vi "createFileInstance.vi"(0 "reference in":refnum<class "File Controller.lvclass">, 2 "TSR?":bool, 3 "TYPE:":string, 5 "error in (no error)":errorcluster) -> (14 "reference out":refnum<class "File Controller.lvclass">, 19 "error out":errorcluster)   [LabVIEW 2015, in "File Controller.lvclass"]
uses:
  File Controller.lvclass
  APP/excelFile_class/fileType.ctl
  APP/excelFile_class/excelFile.lvclass
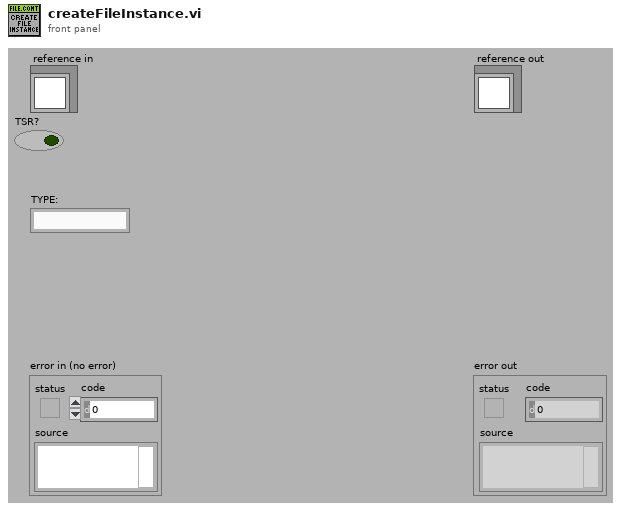
[diagram p1: front panel]
types:
  T1 = typedef "excelFile.lvclass/fileType.ctl" = enum16{"devices", "items", "partsTracking", "TSR"}
  T2 = typedef "File Controller.lvclass/ObjectAttributesRef.ctl" = refnum<data-value>
  T3 = typedef "File Controller.lvclass/ObjectAttributes.ctl" = cluster{"MyAttribute":dbl, "excelFile_refs":refnum<class "excelFile.lvclass">[], "filePaths":path[], "outlookTemplatePaths":path[], "attachmentTemplatePaths":path[], "configFilePath":path, "not_setting":bool[], "python_ref":refnum<class "python.lvclass">, "TSR":cluster{"number":string, "TSR_path":path, "service_path":path}}
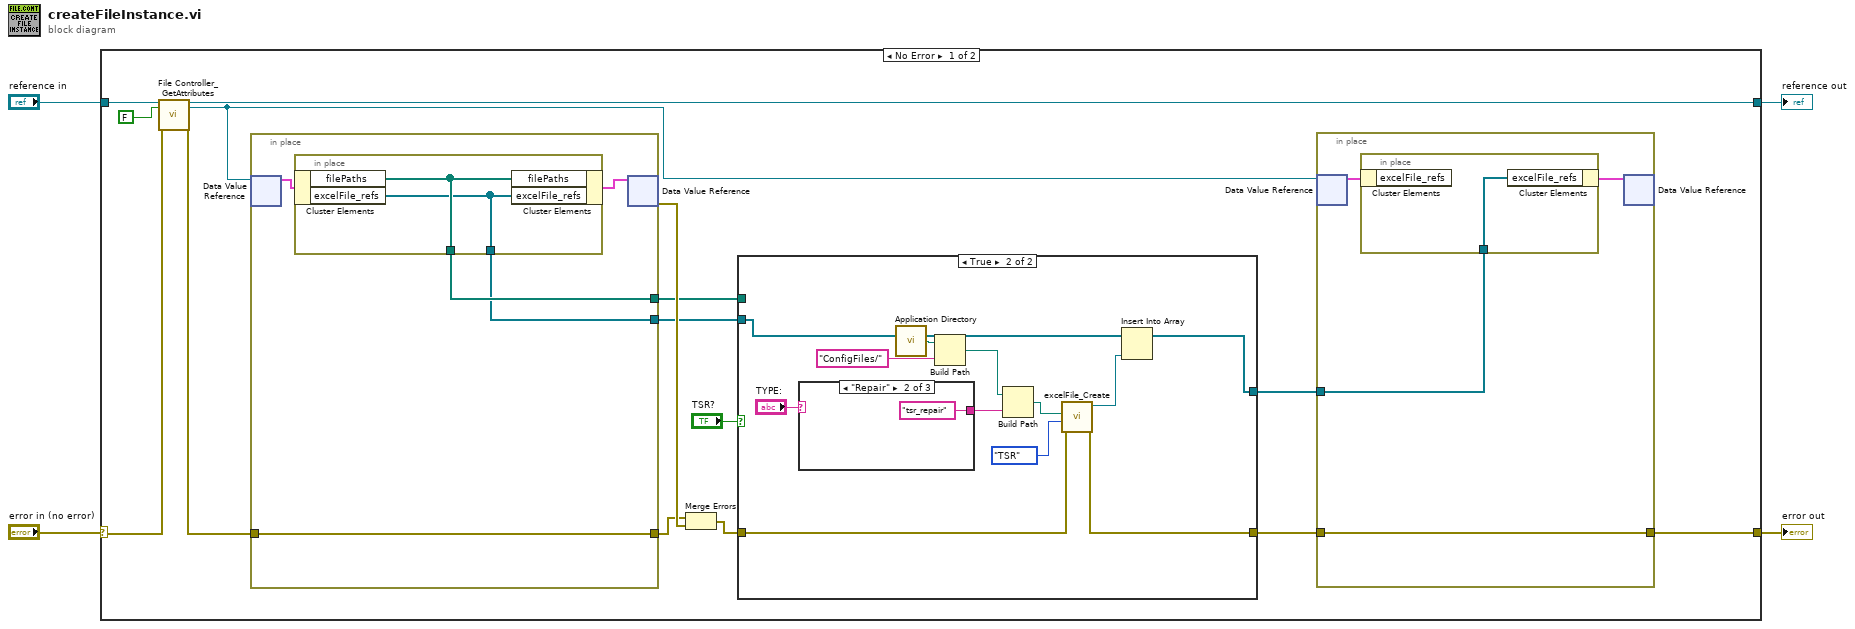
[diagram p0: block diagram]
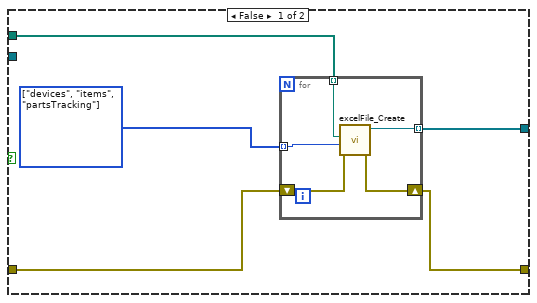
[diagram p2: hidden frame]
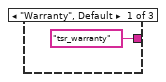
[diagram p3: hidden frame]
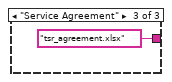
[diagram p4: hidden frame]
diagram:
  n1 = case shown="No Error" "error in (no error)" {
    selector: "error in (no error)" -> [w15 w58]
    tunnel: [w9 w58] -> w3
    tunnel: [w13 w57] -> w1
    tunnel: "reference in" -> [w17 w57]
    frame No Error {
      n2 = call "File Controller_GetAttributes.vi"("reference in"=w17, "return data? (T)"=FALSE, "error in (no error)"=w15) -> ("reference out"=w13:refnum<class "File Controller.lvclass">, "attributes ref"=w8:T2, "error out"=w14:errorcluster)  [unwired: 13 in, 1 out]
      n3 = in-place {
        in-place-border: w14 -> [w52]
        in-place-border: [w52] -> w18
        in-place-border: [w51] -> w11
        in-place-border: [w50] -> w5
        n4 = in-place-dvr #1(w8) -> (w53:T3)  [unwired: 1 out]
        n5 = in-place {
          in-place-border: [w56] -> w51
          in-place-border: [w55] -> w50
          n6 = in-place-cluster #2(w53) -> ("filePaths"=w56:path[], "excelFile_refs"=w55:refnum<class "excelFile.lvclass">[])
          n7 = in-place-cluster #2("filePaths"=w56, "excelFile_refs"=w55) -> (w54:T3)
        }
        n8 = in-place-dvr #1(w54) -> (w19:errorcluster)  [unwired: 1 out]
      }
      n9 = Merge Errors(w18, w19) -> (w12:errorcluster)
      n10 = case shown="True" "TSR?" {
        tunnel: w12 -> [w23 w38]
        tunnel: w11 -> [w22 _]
        tunnel: [w21 w37] -> w10
        tunnel: [w20 w40] -> w7
        tunnel: w5 -> [_ w41]
        frame False {
          w24 = T1[] [enum."devices", enum."items", enum."partsTracking"] items=["devices", "items", "partsTracking", "TSR"]
          n11 = for {
            shift-right: [w26] -> w21
            shift-left: w23 -> [w29]
            tunnel: w24 -> [w28] mode=indexing
            tunnel: w22 -> [w27] mode=indexing
            tunnel: [w25] -> w20 mode=indexing
            n12 = call "excelFile_Create.vi"("error in (no error)"=w29, "fileType"=w28, "Path"=w27) -> ("error out"=w26:errorcluster, "reference out"=w25:refnum<class "excelFile.lvclass">)  [unwired: 7 in]
          }
        }
        frame True {
          n13 = case shown="\"Repair\"" "TYPE:" {
            tunnel: ["tsr_warranty" ("name or relative path") "tsr_repair" ("name or relative path") "tsr_agreement.xlsx" ("name or relative path")] -> w34
            frame "Warranty", Default {
            }
            frame "Repair" {
            }
            frame "Service Agreement" {
            }
          }
          n14 = call <vilib>:"Application Directory.vi"() -> ("Application Directory"=w31:path)
          n15 = Build Path(base path=w31, name or relative path="ConfigFiles/") -> (appended path=w33:path)
          n16 = Build Path(base path=w33, name or relative path=w34) -> (appended path=w30:path)
          n17 = call "excelFile_Create.vi"("error in (no error)"=w38, "fileType"=fileType."TSR", "Path"=w30) -> ("error out"=w37:errorcluster, "reference out"=w39:refnum<class "excelFile.lvclass">)  [unwired: 7 in]
          n18 = Insert Into Array(array=w41, new element=w39) -> (w40:refnum<class "excelFile.lvclass">[])  [unwired: 1 in]
        }
      }
      n19 = in-place {
        in-place-border: w10 -> [w46]
        in-place-border: [w46] -> w9
        in-place-border: w7 -> [w45]
        n20 = in-place-dvr #3(w8) -> (w47:T3)  [unwired: 1 out]
        n21 = in-place {
          in-place-border: w45 -> [w49]
          n22 = in-place-cluster #4(w47) -> ()  [unwired: 1 out]
          n23 = in-place-cluster #4("excelFile_refs"=w49) -> (w48:T3)
        }
        n24 = in-place-dvr #3(w48) -> ()  [unwired: 2 out]
      }
    }
    frame Error {
    }
  }
  "error out" <- w3
  "reference out" <- w1
